vi "Create Send Message Policy.vi"(8 "error in (no error)":errorcluster, 10 "Role Name":string, 11 "SQS in":refnum<class "Queue.lvclass">) -> (0 "error out":errorcluster, 3 "SQS out":refnum<class "Queue.lvclass">)   [LabVIEW 2015, in "NI_AWS_SQS.lvlib" / "Queue.lvclass"]
uses:
  Queue.lvclass
  Queue Attribute.ctl
  Queue.lvclass/Queue.ctl
  Core/HTTP Request/HTTP Request.lvclass/HTTP Request.ctl
  Read Name.vi
  Core/HTTP Request/Read Credentials.vi
  IAM/IAM Session/IAM Session.lvclass
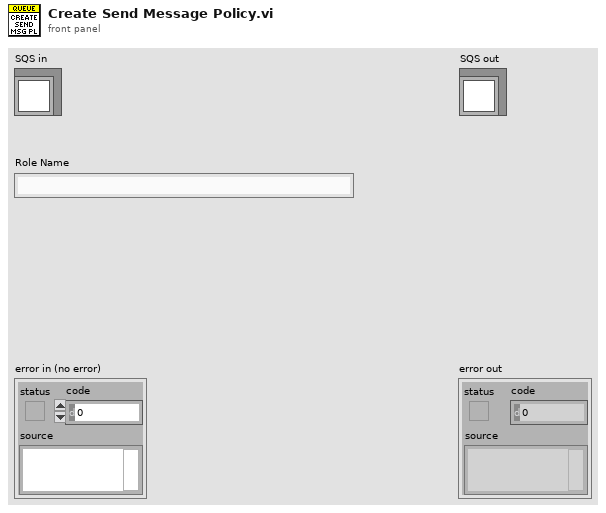
[diagram p1: front panel]
types:
  T1 = typedef "NI_AWS_SQS.lvlib/Queue.lvclass/Queue Attribute Value Pair.ctl" = cluster{"Attribute":T2, "Value":string}
  T2 = typedef "NI_AWS_SQS.lvlib/Queue.lvclass/Queue Attribute.ctl" = enum16{"ApproximateNumberOfMessages", "ApproximateNumberOfMessagesDelayed", "ApproximateNumberOfMessagesNotVisible", "CreatedTimestamp", "DelaySeconds", "LastModifiedTimestamp", "MaximumMessageSize", "MessageRetentionPeriod", "Policy", "QueueArn", "ReceiveMessageWaitTimeSeconds", "RedrivePolicy", "VisibilityTimeout"}
  T3 = typedef "NI_AWS_Core.lvlib/HTTP Request.lvclass/AWS Credentials.ctl" = cluster{"Access Key":string, "Secret Key":string}
  T4 = typedef "NI_AWS_IAM.lvlib/Policy.ctl" = cluster{"Name":string, "Default Version ID":string, "ID":string, "Path":string, "ARN":string, "Attachment Count":i32, "Creation Date":string, "Last Updated Date":string}
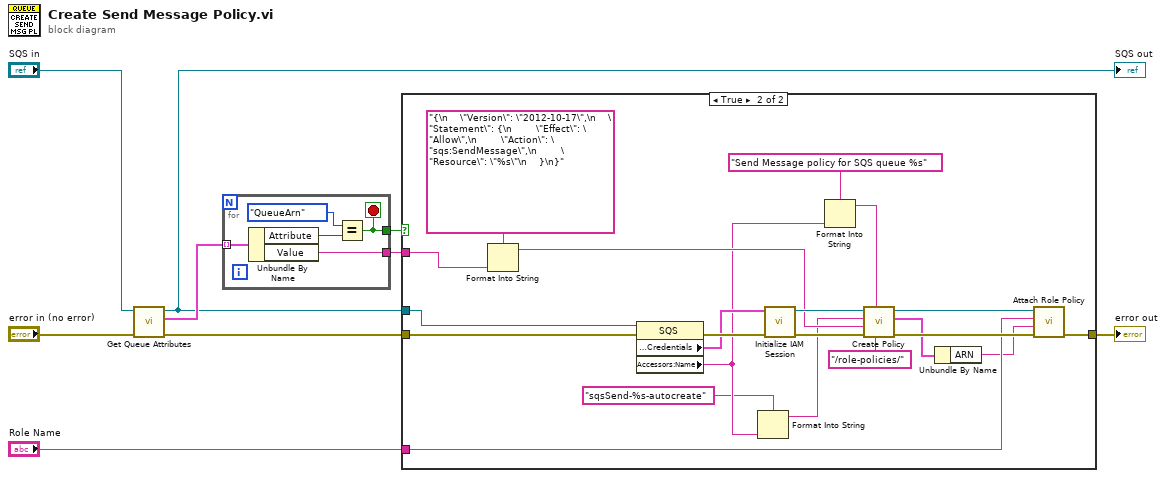
[diagram p0: block diagram]
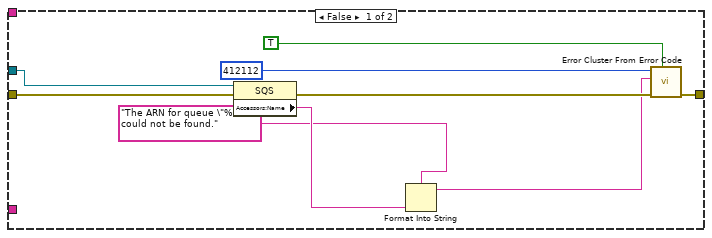
[diagram p2: hidden frame]
diagram:
  n1 = call "Get Queue Attributes.vi"("error in (no error)"="error in (no error)", "SQS in"="SQS in") -> ("error out"=w6:errorcluster, "Attribute Results"=w7:T1[], "SQS out"=w2:refnum<class "Queue.lvclass">)  [unwired: 7 in]
  "SQS out" <- w2
  n2 = for {
    tunnel: w7 -> [w14] mode=indexing
    tunnel: [w13] -> w4
    tunnel: [w10] -> w5
    stop <- w10 stop-if-true
    n3 = Unbundle By Name(w14) -> ("Attribute"=w12:T2, "Value"=w13:string)
    n4 = Equal?(x=Queue_Attribute."QueueArn", y=w12) -> (x = y?=w10:bool)
  }
  n5 = case shown="True" w5 {
    tunnel: w6 -> [w23 w44]
    tunnel: w4 -> [_ w28]
    tunnel: [w22 w30] -> w3
    tunnel: w2 -> [w20 w43]
    tunnel: "Role Name" -> [_ w33]
    frame False {
      n6 = property class="SQS"(reference=w20, error in=w23) -> (error out=w21:errorcluster, "Accessors:Name"=w19:string)  [unwired: 1 out]
      n7 = Format Into String(format string="The ARN for queue \"%s\" could not be found.", w19) -> (resulting string=w17:string)  [unwired: 2 in, 1 out]
      n8 = call <vilib>:"Error Cluster From Error Code.vi"("show call chain? (False)"=TRUE, "error in (no error)"=w21, "error message (\"\")"=w17, "error code (0)"=412112) -> ("error out"=w22:errorcluster)  [unwired: 5 in]
    }
    frame True {
      n9 = Format Into String(format string="{\n    \"Version\": \"2012-10-17\",\n    \"Statement\": {\n        \"Effect\": \"Allow\",\n        \"Action\": \"sqs:SendMessage\",\n        \"Resource\": \"%s\"\n    }\n}", w28) -> (resulting string=w27:string)  [unwired: 2 in, 1 out]
      n10 = property class="SQS"(reference=w43, error in=w44) -> (error out=w42:errorcluster, "Accessors:Credentials"=w41:T3, "Accessors:Name"=w26:string)  [unwired: 1 out]
      n11 = Format Into String(format string="sqsSend-%s-autocreate", w26) -> (resulting string=w24:string)  [unwired: 2 in, 1 out]
      n12 = call "Initialize IAM Session.vi"("error in (no error)"=w42, "AWS Credentials"=w41) -> ("error out"=w40:errorcluster, "IAM Session"=w39:refnum<class "IAM Session.lvclass">)  [unwired: 8 in]
      n13 = Format Into String(format string="Send Message policy for SQS queue %s", w26) -> (resulting string=w35:string)  [unwired: 2 in, 1 out]
      n14 = call "Create Policy.vi"("Path"="/role-policies/", "Description"=w35, "error in (no error)"=w40, "Document"=w27, "Name"=w24, "IAM Session in"=w39) -> ("error out"=w38:errorcluster, "Created Policy"=w32:T4, "IAM Session out"=w37:refnum<class "IAM Session.lvclass">)  [unwired: 3 in]
      n15 = Unbundle By Name(w32) -> ("ARN"=w31:string)
      n16 = call "Attach Role Policy.vi"("error in (no error)"=w38, "Policy ARN"=w31, "Role Name"=w33, "IAM Session in"=w37) -> ("error out"=w30:errorcluster)  [unwired: 6 in, 1 out]
    }
  }
  "error out" <- w3
